vi "ScaleandControl.vi"(1 "button info":T2, 2 "axis info":T1) -> (0 "String":string)   [LabVIEW 2010]
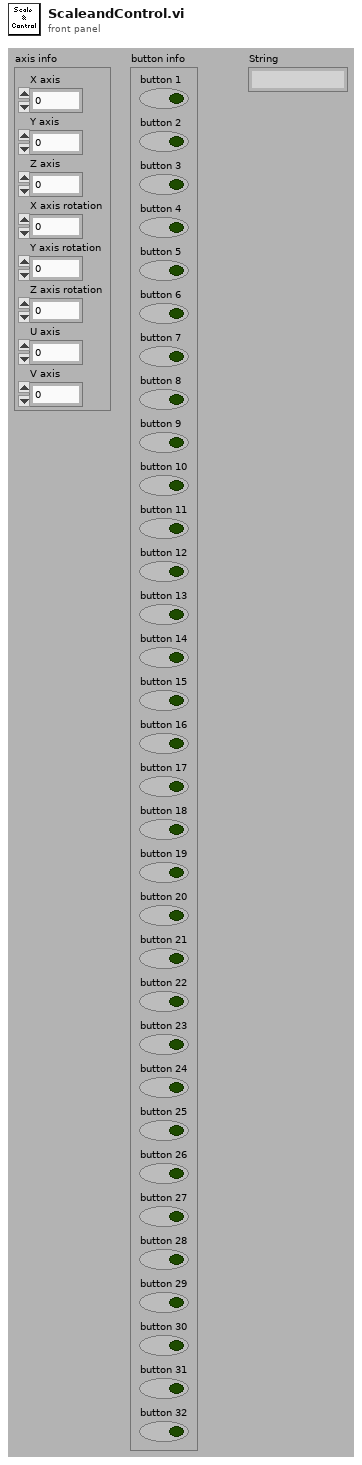
[diagram p1: front panel]
types:
  T1 = cluster{"X axis":i32, "Y axis":i32, "Z axis":i32, "X axis rotation":i32, "Y axis rotation":i32, "Z axis rotation":i32, "U axis":i32, "V axis":i32}
  T2 = cluster{"button 1":bool, "button 2":bool, "button 3":bool, "button 4":bool, "button 5":bool, "button 6":bool, "button 7":bool, "button 8":bool, "button 9":bool, "button 10":bool, "button 11":bool, "button 12":bool, "button 13":bool, "button 14":bool, "button 15":bool, "button 16":bool, "button 17":bool, "button 18":bool, "button 19":bool, "button 20":bool, "button 21":bool, "button 22":bool, "button 23":bool, "button 24":bool, "button 25":bool, "button 26":bool, "button 27":bool, "button 28":bool, "button 29":bool, "button 30":bool, "button 31":bool, "button 32":bool}
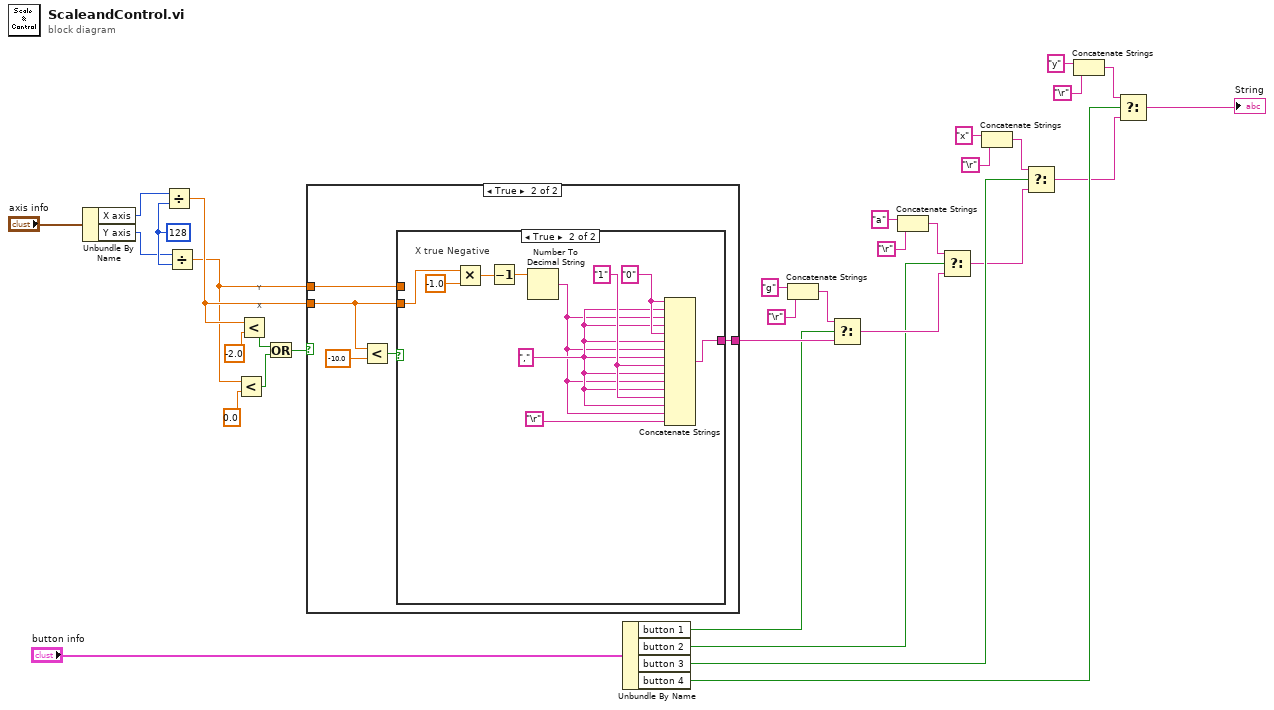
[diagram p0: block diagram]
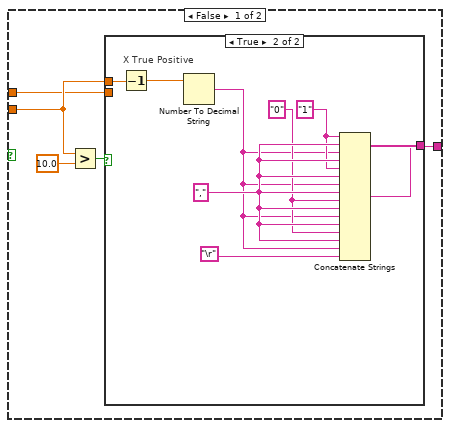
[diagram p2: hidden frame]
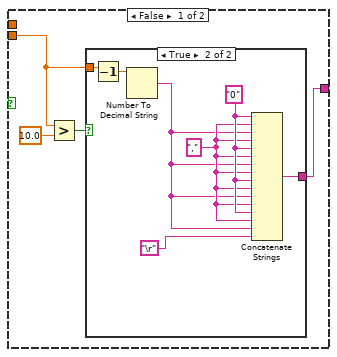
[diagram p3: hidden frame]
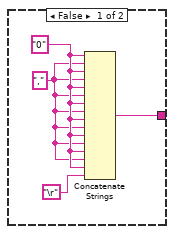
[diagram p4: hidden frame]
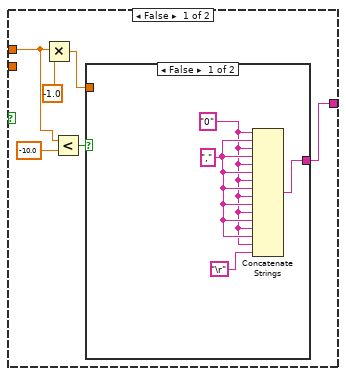
[diagram p5: hidden frame]
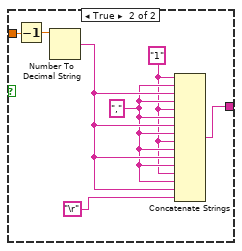
[diagram p6: hidden frame]
diagram:
  w24 = 128 ("y")
  # "X"
  # "Y"
  n1 = Unbundle By Name("axis info") -> ("X axis"=w22:i32, "Y axis"=w21:i32)
  n2 = Divide(x=w22, y=w24) -> (x/y=w27:dbl)
  n3 = Divide(x=w21, y=w24) -> (x/y=w20:dbl)
  n4 = Less?(x=w20, y=0.0) -> (x < y?=w26:bool)
  n5 = Less?(x=w27, y=-2.0) -> (x < y?=w29:bool)
  n6 = Or(x=w29, y=w26) -> (x .or. y?=w25:bool)
  n7 = case shown="True" w25 {
    tunnel: [w36 w64] -> w7
    tunnel: w27 -> [w35 w63]
    tunnel: w20 -> [w34 w62]
    frame False {
      n8 = Greater?(x=w35, y=10.0) -> (0:w38:bool)
      n9 = case shown="True" w38 {
        tunnel: [w40 w55] -> w36
        tunnel: w35 -> [_ w61]
        tunnel: w34 -> [w39 _]
        frame False {
          n10 = Greater?(x=w39, y=10.0) -> (0:w41:bool)
          n11 = case shown="True" w41 {
            tunnel: [w43 w53] -> w40
            tunnel: w39 -> [_ w52]
            frame False {
              w44 = "," ("string")
              w45 = "0" ("string")
              n12 = Concatenate Strings(w45, w44, w45, w44, w45, w44, w45, w44, w45, w44, w45, w44, w45, w44, w45, "\r") -> (w43:string)
            }
            frame True {
              w48 = "," ("string")
              w49 = "0" ("string")
              n13 = Decrement(x=w52) -> (x-1=w51:dbl)
              n14 = Number To Decimal String(number=w51) -> (decimal integer string=w47:string)  [unwired: 1 in]
              n15 = Concatenate Strings(w49, w48, w47, w48, w49, w48, w47, w48, w49, w48, w47, w48, w49, w48, w47, "\r") -> (w53:string)
            }
          }
        }
        frame True {
          w57 = "0" ("string")
          w56 = "1" ("string")
          w59 = "," ("string")
          # "X True Positive"
          n16 = Decrement(x=w61) -> (x-1=w60:dbl)
          n17 = Number To Decimal String(number=w60) -> (decimal integer string=w54:string)  [unwired: 1 in]
          n18 = Concatenate Strings(w56, w59, w54, w59, w56, w59, w54, w59, w57, w59, w54, w59, w57, w59, w54, "\r") -> (w55:string)
        }
      }
    }
    frame True {
      n19 = Less?(x=w63, y=-10.0) -> (x < y?=w66:bool)
      n20 = case shown="True" w66 {
        tunnel: [w70 w85] -> w64
        tunnel: w63 -> [_ w92]
        tunnel: w62 -> [w67 _]
        frame False {
          n21 = Multiply(x=w67, y=-1.0) -> (x*y=w68:dbl)
          n22 = Less?(x=w67, y=-10.0) -> (x < y?=w71:bool)
          n23 = case shown="False" w71 {
            tunnel: [w76 w78] -> w70
            tunnel: w68 -> [_ w77]
            frame False {
              w75 = "," ("string")
              w74 = "0" ("string")
              n24 = Concatenate Strings(w74, w75, w74, w75, w74, w75, w74, w75, w74, w75, w74, w75, w74, w75, w74, "\r") -> (w76:string)
            }
            frame True {
              w82 = "," ("string")
              w81 = "1" ("string")
              n25 = Decrement(x=w77) -> (x-1=w79:dbl)
              n26 = Number To Decimal String(number=w79) -> (decimal integer string=w83:string)  [unwired: 1 in]
              n27 = Concatenate Strings(w81, w82, w83, w82, w81, w82, w83, w82, w81, w82, w83, w82, w81, w82, w83, "\r") -> (w78:string)
            }
          }
        }
        frame True {
          w88 = "1" ("string")
          w89 = "0" ("string")
          w86 = "," ("string")
          # "X true Negative"
          n28 = Multiply(x=w92, y=-1.0) -> (x*y=w91:dbl)
          n29 = Decrement(x=w91) -> (x-1=w90:dbl)
          n30 = Number To Decimal String(number=w90) -> (decimal integer string=w84:string)  [unwired: 1 in]
          n31 = Concatenate Strings(w89, w86, w84, w86, w89, w86, w84, w86, w88, w86, w84, w86, w88, w86, w84, "\r") -> (w85:string)
        }
      }
    }
  }
  n32 = Unbundle By Name("button info") -> ("button 1"=w6:bool, "button 2"=w5:bool, "button 3"=w4:bool, "button 4"=w3:bool)
  n33 = Concatenate Strings("g" ("string"), "\r") -> (w33:string)
  n34 = Select(t=w33, s=w6, f=w7) -> (s? t:f=w9:string)
  n35 = Concatenate Strings("a" ("string"), "\r") -> (w18:string)
  n36 = Select(t=w18, s=w5, f=w9) -> (s? t:f=w2:string)
  n37 = Concatenate Strings("x" ("string"), "\r") -> (w15:string)
  n38 = Select(t=w15, s=w4, f=w2) -> (s? t:f=w1:string)
  n39 = Concatenate Strings("y" ("string"), "\r") -> (w12:string)
  n40 = Select(t=w12, s=w3, f=w1) -> (s? t:f=→"String":string)
